vi "1-pointcal-v2.vi"() -> ()   [LabVIEW 2018]
uses:
  <vilib>/Utility/NIReport.llb/NI_report.lvclass
  <vilib>/Utility/NIReport.llb/Excel/NI_Excel.lvclass
  <vilib>/Utility/NIReport.llb/Report Type.ctl
  <vilib>/DAQmx/read.llb/DAQmx Read (Analog Wfm 1Chan NSamp).vi
  <vilib>/Utility/NIReport.llb/Append Text Table to Report (wrap).vi
  <vilib>/Utility/NIReport.llb/Append Numeric Table to Report (wrap).vi
  <vilib>/DAQmx/create/channels.llb/DAQmx Create Channel (AI-Voltage-Basic).vi
  <vilib>/DAQmx/configure/timing.llb/DAQmx Timing (Sample Clock).vi
  <vilib>/DAQmx/miscellaneous.llb/DAQmx Fill In Error Info.vi
  <vilib>/Utility/NIReport.llb/NI_ReportGenerationCore.lvlib
  <resource>/objmgr/daqmx.rc
panel:
  in  "Unit":enum16{"oz.in", "lbf-ft.", "lbf-in.", "N-m"}(ring)
  in  "Sensor ID:":tag
  in  "samples per channel":i32=4000
  in  "rate":dbl=500.0 format="%#_13g"
  in  "milliseconds to wait":u32=1000
  out "Cycles":i32=10
  out "Average":dbl[](array[numeric])=[2.9362440950071025]
  out "Template":refnum<class "NI_report.lvclass">
  out "Upper Limit":dbl=2.12
  out "Lower Limit":dbl=1.88
  out "output array":dbl[][](array[numeric])=[[3.9379769276696557, 2.0, 2.0, 3.7231645789771317, 3.939138075500426], [2.0, 2.0, 3.7939945966541258, 3.968166771269686, 2.0]]
  in  "stop":bool
  out "Torque":dbl=3.9379769276696557 format="%0.2f"
  out "Waveform Graph 2":waveform(dbl)(graph)={"t0"=timestamp(3654803301.2825823 s since 1904-01-01), "dt"=0.000333325, "Y"=array[6000 elements], "attributes"=variant("NI_ChannelName"=variant(string "6003/ai0"), "NI_UnitDescription"=variant(string "oz.in"))}
  in  "Continue":bool=TRUE
  out "Torque:":dbl=2.0
  in  "Humidity(%):":string="40"
  in  "Temp(F):":string="75"
  in  "FG Serial Number:":string="0211932-0056"
  in  "User Name:":string="Kyle Watts"
  in  "FG Model:":string(combo)="FG-40i"
  in  "Cal Dir:":string(combo)="CW"
  # "Calibration Tester"
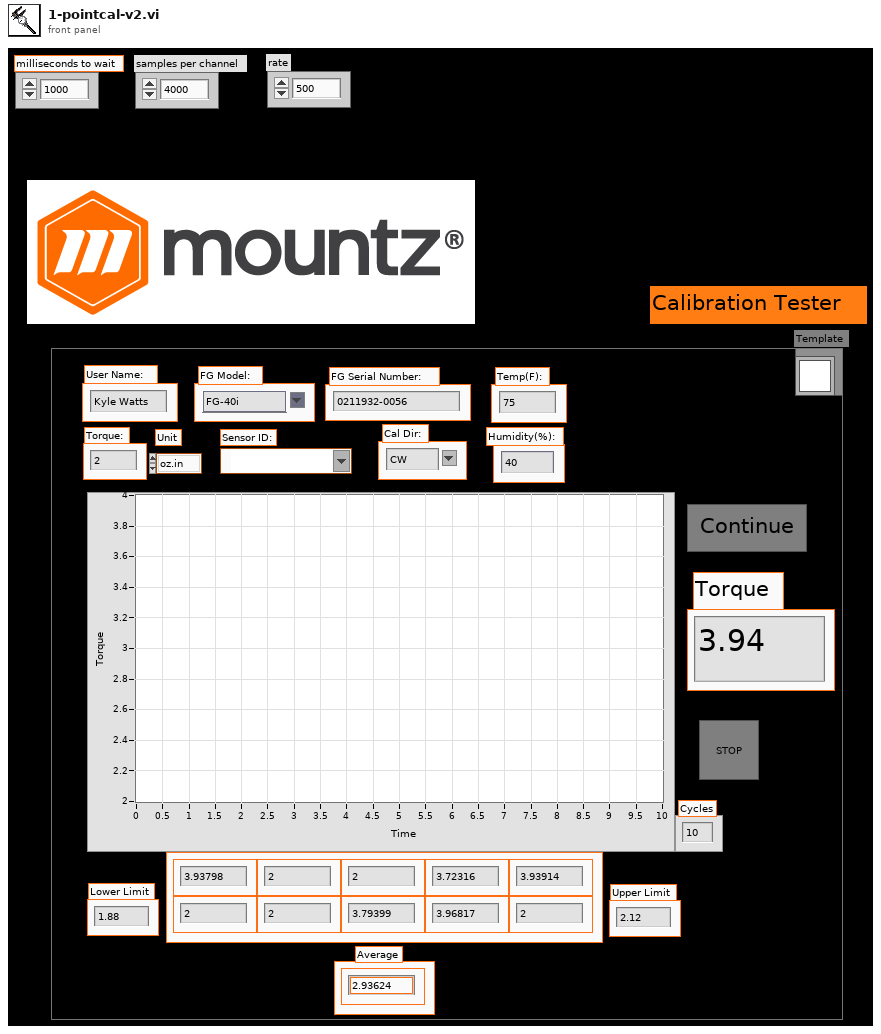
[diagram p1: front panel]
types:
  T1 = enum16{"Initialize ", "Set Torque", "Read Torque"}
  T2 = enum16{"Initialize ", "Set Torque", "Read Torque", "Save data"}
  T3 = cluster{"position (excel)":cluster{"row":i32, "column":i32}, "name (excel)":string, "bookmark (word)":string}
  T4 = cluster{"Charset (-1)":i16, "Weight (-1)":i16, "Name":string, "Size":string}
  T5 = typedef "NI_ReportGenerationCore.lvlib/Report Type.ctl" = enum16{"HTML", "Word", "Excel"}
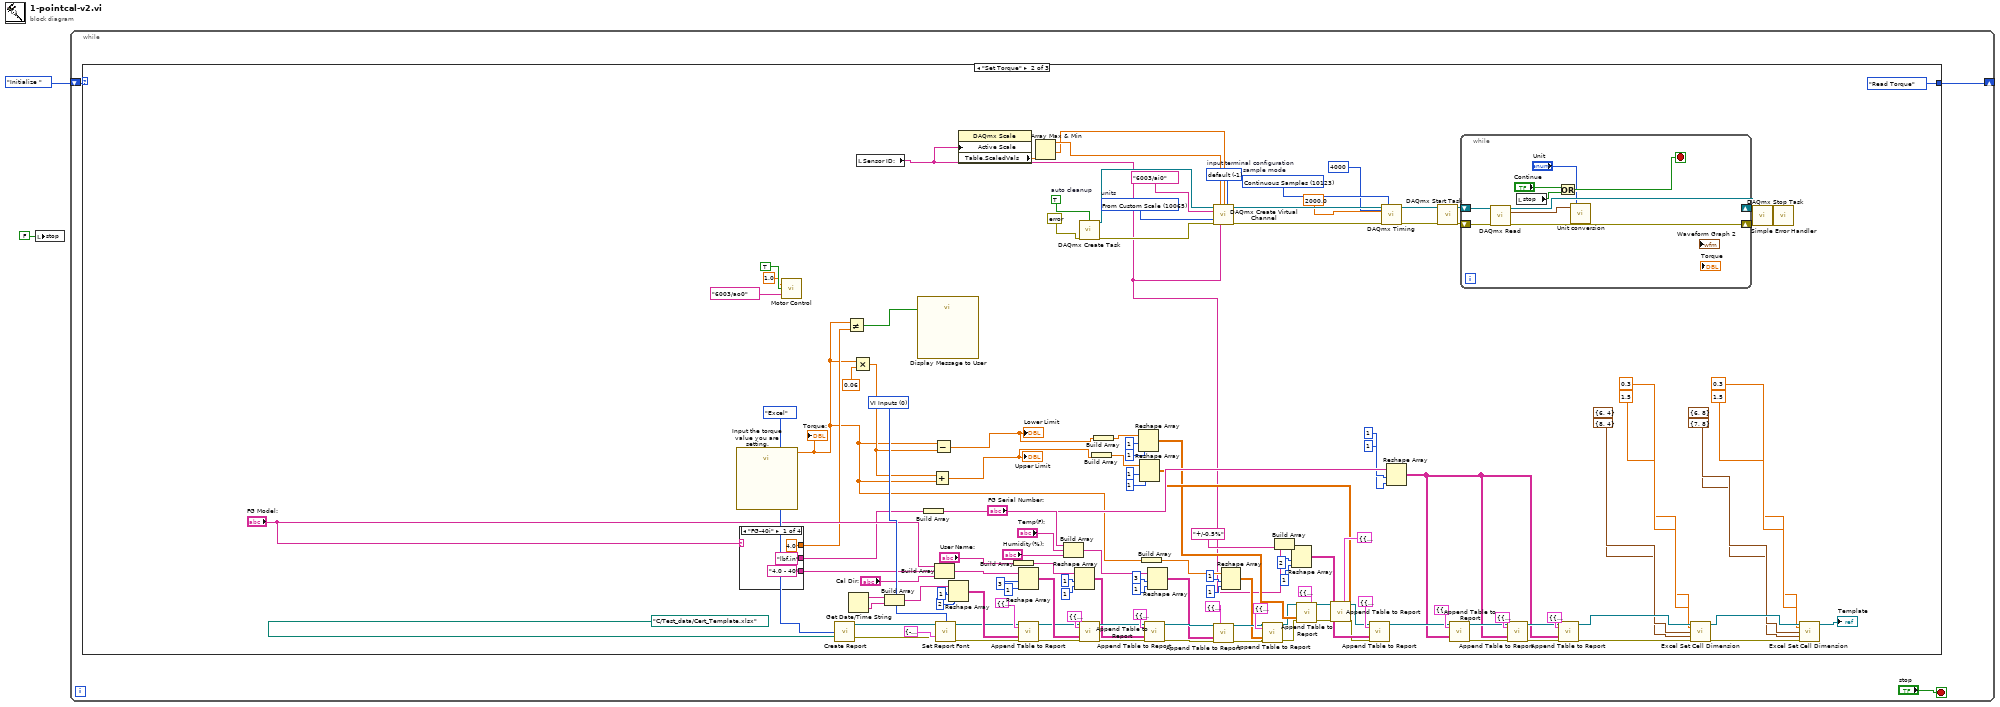
[diagram p0: block diagram]
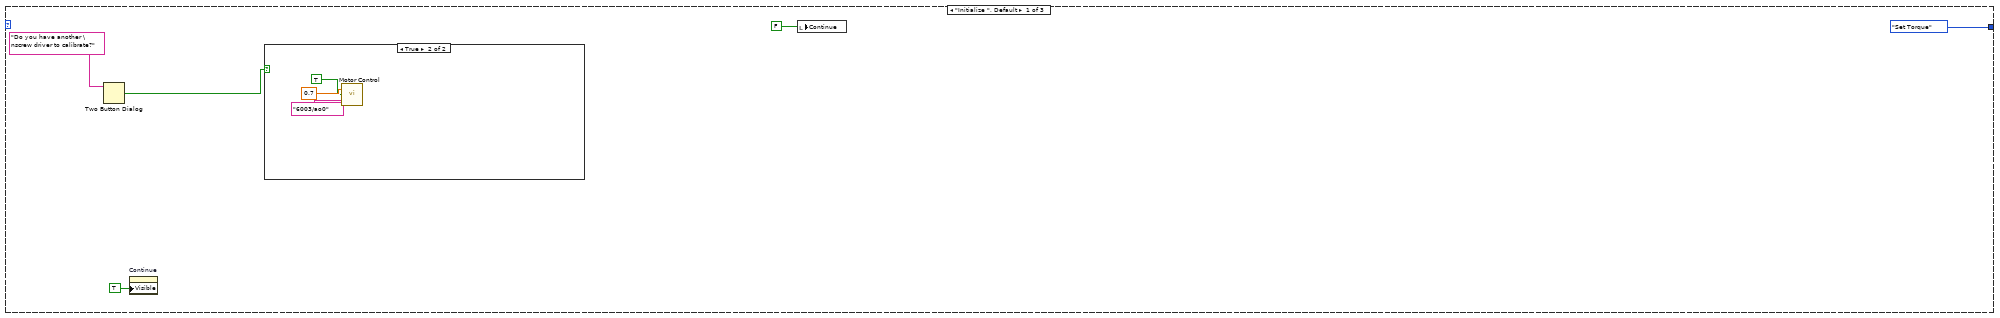
[diagram p2: hidden frame]
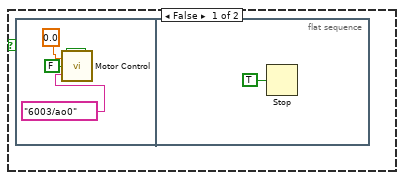
[diagram p3: hidden frame]
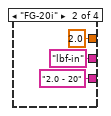
[diagram p4: hidden frame]
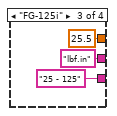
[diagram p5: hidden frame]
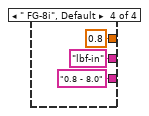
[diagram p6: hidden frame]
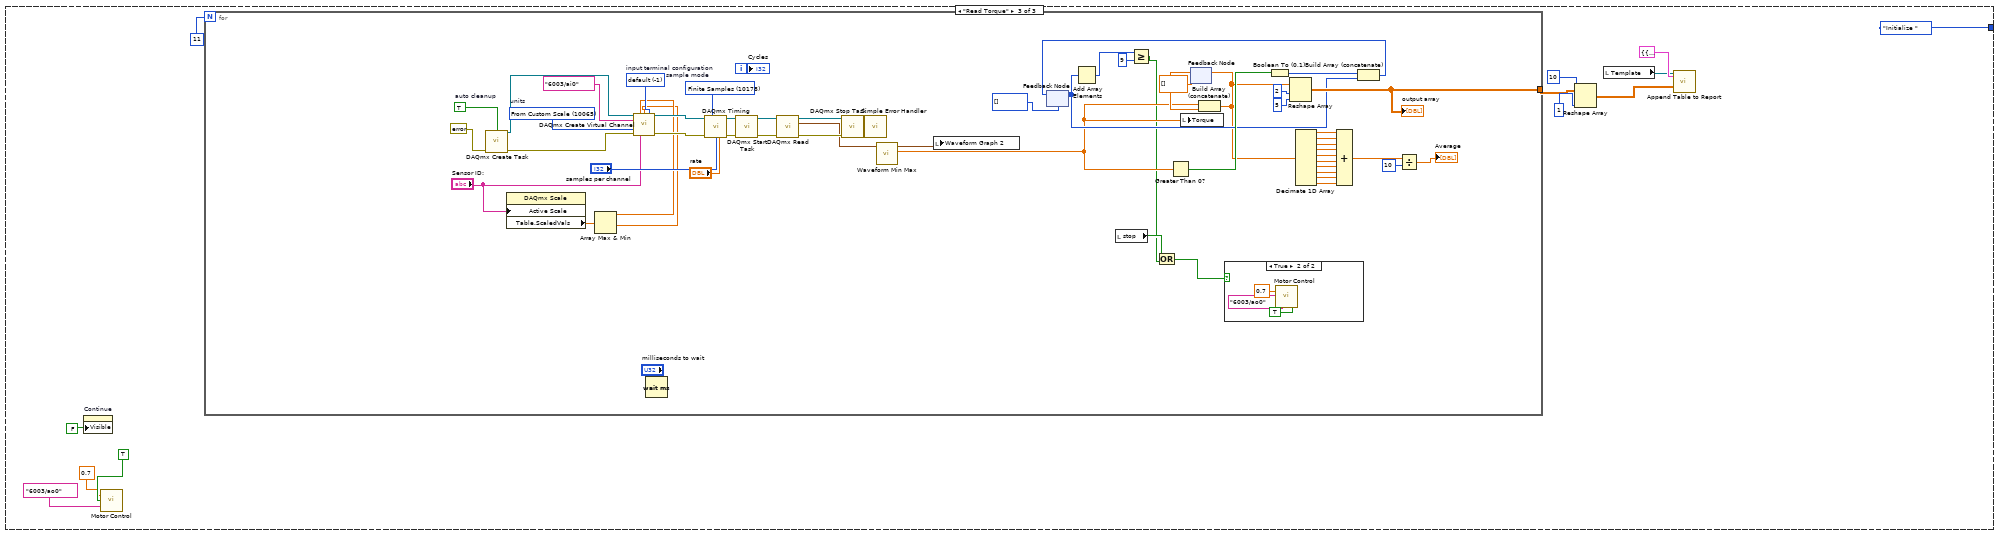
[diagram p7: hidden frame]
diagram:
  n1 = local write "stop"(FALSE ("stop")) -> ()
  n2 = while {
    shift-right: [w3] -> _
    shift-left: T1."Initialize " -> [w4]
    stop <- "stop" stop-if-true
    n3 = case shown="\"Set Torque\"" w4 {
      tunnel: [T2."Set Torque" T2."Read Torque" T2."Initialize "] -> w3
      frame "Initialize ", Default {
        n4 = Two Button Dialog(message="Do you have another \nscrew driver to calibrate?") -> (T button?=w6:bool)  [unwired: 2 in]
        n5 = property on="Continue" class="Bool (strict)"("Visible"=TRUE) -> ()  [unwired: 2 in, 2 out]
        n6 = case shown="True" w6 {
          frame False {
            n7 = flat-sequence {
              frame #0 {
                n8 = call "Motor Control.vi"("Run"=FALSE, "physical channels"=tag "6003/ao0", "Speed"=0.0) -> ()
              }
              frame #1 {
                n9 = Stop(stop? (T)=TRUE) -> ()
              }
            }
          }
          frame True {
            n10 = call "Motor Control.vi"("Run"=TRUE, "physical channels"=tag "6003/ao0", "Speed"=0.7) -> ()
          }
        }
        n11 = local write "Continue"(FALSE ("Continue")) -> ()
      }
      frame "Set Torque" {
        w54 = 10123 items=["Finite Samples"=10178, "Continuous Samples"=10123, "Hardware Timed Single Point"=12522]  # sample mode
        w52 = -1 items=["default"=-1, "RSE"=10083, "NRSE"=10078, "Differential"=10106, "Pseudodifferential"=12529]  # input terminal configuration
        w51 = 10065 items=["Volts"=10348, "From Custom Scale"=10065]  # units
        w48 = TRUE  # auto cleanup
        w120 = u16 0 items=["VI Inputs", "Font Dialog Box"] ("font settings source (VI Inputs)")
        n12 = call "Input the torque value you are setting."() -> ("Torque"=w63:dbl)  [unwired: 17 in, 2 out]
        "Torque:" <- w63
        n13 = case shown="\"FG-40i\"" "FG Model:" {
          tunnel: ["4.0 - 40" "2.0 - 20" "25 - 125" "0.8 - 8.0"] -> w99
          tunnel: ["lbf.in" "lbf-in" "lbf.in" "lbf-in"] -> w70
          tunnel: [4.0 2.0 25.5 0.8] -> w68
          frame "FG-40i" {
          }
          frame "FG-20i" {
          }
          frame "FG-125i" {
          }
          frame " FG-8i", Default {
          }
        }
        n14 = call "Motor Control.vi"("Run"=TRUE, "physical channels"=tag "6003/ao0", "Speed"=1.0) -> ()
        n15 = call <vilib>:"Create Report.vi"("report type"=Report_Type."Excel", "template (empty)"=path "C:/Test_data/Cert_Template.xlsx") -> ("report out"=w119:refnum<class "NI_report.lvclass">, "error out"=w118:errorcluster)  [unwired: 12 in]
        n16 = Not Equal?(x=w63, y=w68) -> (x != y?=w67:bool)
        n17 = Get Date/Time String() -> (date string=w137:string, time string=w138:string)  [unwired: 3 in]
        n18 = Multiply(x=w63, y=0.06) -> (x*y=w64:dbl)
        n19 = local read "Sensor ID:"() -> (w21:tag)
        n20 = Build Array(w137, w138) -> (w141:string[])
        n21 = call "Display Message to User"("Enable"=w67) -> ()  [unwired: 9 in, 2 out]
        n22 = Build Array(w70) -> (w73:string[])
        n23 = Add(x=w64, y=w63) -> (x+y=w30:dbl)
        "Upper Limit" <- w30
        n24 = Subtract(x=w63, y=w64) -> (x-y=w31:dbl)
        "Lower Limit" <- w31
        n25 = Build Array("FG Model:", w99, "Cal Dir:") -> (w101:string[])
        n26 = call-dynamic "Set Report Font.vi"("report in"=w119, "font settings source (VI Inputs)"=w120, "font settings"=T4 {"Charset (-1)"=-1, "Weight (-1)"=-1, "Name"="Calibri", "Size"=" 14"}, "error in (no error)"=w118) -> ("report out"=w116:refnum<class "NI_report.lvclass">, "error out"=w117:errorcluster)  [unwired: 9 in, 1 out]
        n27 = Reshape Array(w141, 1 ("dimension size"), 2 ("dimension size")) -> (w140:string[][])
        n28 = property class="DAQmx Scale"("Active Scale"=w21) -> ("Table.ScaledVals"=w20:dbl[])  [unwired: 2 in, 2 out]
        n29 = Build Array("User Name:") -> (w94:string[])
        n30 = Reshape Array(w101, 3 ("dimension size"), 1 ("dimension size")) -> (w100:string[][])
        n31 = call-poly <vilib>:"Append Table to Report.vi"("report in"=w116, "MS Office parameters"=T3 {"position (excel)"={"row"=4, "column"=8}, "name (excel)"="", "bookmark (word)"=""}, "text data"=w140, "error in (no error)"=w117) -> ("report out"=w96:refnum<class "NI_report.lvclass">, "error out"=w95:errorcluster)  [unwired: 8 in, 2 out]
        n32 = Array Max & Min(array=w20) -> (max value=w19:dbl, min value=w18:dbl)  [unwired: 2 out]
        n33 = Build Array("FG Serial Number:", "Temp(F):", "Humidity(%):") -> (w89:string[])
        n34 = Reshape Array(w94, 1 ("dimension size"), 1 ("dimension size")) -> (w90:string[][])
        n35 = call <vilib>:"DAQmx Create Task.vi"("auto cleanup"=w48, "error in"=errorcluster {"status"=FALSE, "code"=0, "source"=""}) -> ("task out"=w49:refnum<k21>, "error out"=w47:errorcluster)  [unwired: 12 in]
        n36 = call-poly <vilib>:"Append Table to Report.vi"("report in"=w96, "MS Office parameters"=T3 {"position (excel)"={"row"=5, "column"=1}, "name (excel)"="", "bookmark (word)"=""}, "text data"=w100, "error in (no error)"=w95) -> ("report out"=w131:refnum<class "NI_report.lvclass">, "error out"=w132:errorcluster)  [unwired: 8 in, 2 out]
        n37 = Build Array(w30) -> (w32:dbl[])
        n38 = Build Array(w31) -> (w33:dbl[])
        n39 = Reshape Array(w33, 1 ("dimension size"), 1 ("dimension size")) -> (w28:dbl[][])
        n40 = Reshape Array(w32, 1 ("dimension size"), 1 ("dimension size")) -> (w29:dbl[][])
        n41 = Build Array(w63) -> (w82:dbl[])
        n42 = call-poly <vilib>:"Append Table to Report.vi"("report in"=w131, "MS Office parameters"=T3 {"position (excel)"={"row"=5, "column"=4}, "name (excel)"="", "bookmark (word)"=""}, "text data"=w90, "error in (no error)"=w132) -> ("report out"=w130:refnum<class "NI_report.lvclass">, "error out"=w129:errorcluster)  [unwired: 8 in, 2 out]
        n43 = Reshape Array(w89, 3 ("dimension size"), 1 ("dimension size")) -> (w83:string[][])
        n44 = call-poly <vilib>:"DAQmx Create Virtual Channel.vi"("task in"=w49, "maximum value"=w19, "minimum value"=w18, "input terminal configuration"=w52, "physical channels"=tag "6003/ai0", "units"=w51, "error in"=w47, "custom scale name"=w21) -> ("task out"=w53:refnum<k21>, "error out"=w50:errorcluster)  [unwired: 6 in]
        n45 = call-poly <vilib>:"Append Table to Report.vi"("report in"=w130, "MS Office parameters"=T3 {"position (excel)"={"row"=5, "column"=8}, "name (excel)"="", "bookmark (word)"=""}, "text data"=w83, "error in (no error)"=w129) -> ("report out"=w127:refnum<class "NI_report.lvclass">, "error out"=w128:errorcluster)  [unwired: 8 in, 2 out]
        n46 = Reshape Array(w82, 1 ("dimension size"), 1 ("dimension size")) -> (w79:dbl[][])
        n47 = call-poly <vilib>:"Append Table to Report.vi"("report in"=w127, "MS Office parameters"=T3 {"position (excel)"={"row"=9, "column"=1}, "name (excel)"="", "bookmark (word)"=""}, "numerical data"=w79, "error in (no error)"=w128) -> ("report out"=w26:refnum<class "NI_report.lvclass">, "error out"=w27:errorcluster)  [unwired: 8 in, 2 out]
        n48 = Build Array(w21, "+/-0.5%") -> (w75:string[])
        n49 = Reshape Array(w75, 2 ("dimension size"), 1 ("dimension size")) -> (w74:string[][])
        n50 = call-poly <vilib>:"Append Table to Report.vi"("report in"=w26, "MS Office parameters"=T3 {"position (excel)"={"row"=9, "column"=4}, "name (excel)"="", "bookmark (word)"=""}, "numerical data"=w28, "error in (no error)"=w27) -> ("report out"=w25:refnum<class "NI_report.lvclass">, "error out"=w24:errorcluster)  [unwired: 8 in, 2 out]
        n51 = call-poly <vilib>:"Append Table to Report.vi"("report in"=w25, "MS Office parameters"=T3 {"position (excel)"={"row"=9, "column"=7}, "name (excel)"="", "bookmark (word)"=""}, "numerical data"=w29, "error in (no error)"=w24) -> ("report out"=w22:refnum<class "NI_report.lvclass">, "error out"=w23:errorcluster)  [unwired: 8 in, 2 out]
        n52 = call-poly <vilib>:"Append Table to Report.vi"("report in"=w22, "MS Office parameters"=T3 {"position (excel)"={"row"=7, "column"=4}, "name (excel)"="", "bookmark (word)"=""}, "text data"=w74, "error in (no error)"=w23) -> ("report out"=w126:refnum<class "NI_report.lvclass">)  [unwired: 8 in, 3 out]
        n53 = call-poly <vilib>:"DAQmx Timing.vi"("task/channels in"=w53, "sample mode"=w54, "samples per channel"=4000, "rate"=2000.0, "error in"=w50) -> ("task out"=w56:refnum<k21>, "error out"=w45:errorcluster)  [unwired: 9 in]
        n54 = Reshape Array(w73, 1 ("index"), 1 ("index")) -> (w69:string[][])
        n55 = call <vilib>:"DAQmx Start Task.vi"("task/channels in"=w56, "error in"=w45) -> ("task out"=w58:refnum<k21>, "error out"=w57:errorcluster)  [unwired: 12 in]
        n56 = call-poly <vilib>:"Append Table to Report.vi"("report in"=w126, "MS Office parameters"=T3 {"position (excel)"={"row"=9, "column"=2}, "name (excel)"="", "bookmark (word)"=""}, "text data"=w69) -> ("report out"=w125:refnum<class "NI_report.lvclass">, "error out"=w124:errorcluster)  [unwired: 9 in, 2 out]
        n57 = while {
          shift-right: [w156] -> w43
          shift-left: w58 -> [w158]
          shift-right: [w155] -> w42
          shift-left: w57 -> [w157]
          stop <- w152 stop-if-true
          n58 = call-poly <vilib>:"DAQmx Read.vi"("task/channels in"=w158, "error in"=w157) -> ("task out"=w156:refnum<k21>, "data"=w151:waveform(dbl), "error out"=w155:errorcluster)  [unwired: 11 in]
          n59 = local read "stop"() -> (w153:bool)
          n60 = Or(x="Continue", y=w153) -> (x .or. y?=w152:bool)
          n61 = call "Unit conversion.vi"("Convert to"="Unit", "Torque in (Nm)"=w151) -> ()  [unwired: 2 in, 2 out]
        }
        n62 = call-poly <vilib>:"Append Table to Report.vi"("report in"=w125, "MS Office parameters"=T3 {"position (excel)"={"row"=9, "column"=5}, "name (excel)"="", "bookmark (word)"=""}, "text data"=w69, "error in (no error)"=w124) -> ("report out"=w122:refnum<class "NI_report.lvclass">, "error out"=w123:errorcluster)  [unwired: 8 in, 2 out]
        n63 = call-poly <vilib>:"Append Table to Report.vi"("report in"=w122, "MS Office parameters"=T3 {"position (excel)"={"row"=9, "column"=8}, "name (excel)"="", "bookmark (word)"=""}, "text data"=w69, "error in (no error)"=w123) -> ("report out"=w115:refnum<class "NI_report.lvclass">, "error out"=w114:errorcluster)  [unwired: 8 in, 2 out]
        n64 = call <vilib>:"Excel Set Cell Dimension.vi"("report in"=w115, "width (-1)"=1.5, "height (-1)"=0.3, "start (-1, -1)"=cluster{"row":i32, "column":i32} {"row"=6, "column"=4}, "end (-1, -1)"=cluster{"row":i32, "column":i32} {"row"=8, "column"=4}, "error in (no error)"=w114) -> ("report out"=w109:refnum<class "NI_report.lvclass">, "error out"=w108:errorcluster)  [unwired: 8 in]
        n65 = call <vilib>:"DAQmx Stop Task.vi"("task/channels in"=w43, "error in"=w42) -> ("error out"=w41:errorcluster)  [unwired: 12 in, 1 out]
        n66 = call <vilib>:"Simple Error Handler.vi"("error in (no error)"=w41) -> ()  [unwired: 4 in, 5 out]
        n67 = call <vilib>:"Excel Set Cell Dimension.vi"("report in"=w109, "width (-1)"=1.5, "height (-1)"=0.3, "start (-1, -1)"=cluster{"row":i32, "column":i32} {"row"=6, "column"=8}, "end (-1, -1)"=cluster{"row":i32, "column":i32} {"row"=7, "column"=8}, "error in (no error)"=w108) -> ("report out"=→"Template":refnum<class "NI_report.lvclass">)  [unwired: 8 in, 1 out]
      }
      frame "Read Torque" {
        n68 = property on="Continue" class="Bool (strict)"("Visible"=FALSE) -> ()  [unwired: 2 in, 2 out]
        n69 = call "Motor Control.vi"("Run"=TRUE, "physical channels"=tag "6003/ao0", "Speed"=0.7) -> ()
        n70 = for {
          N: 11 -> [_]
          tunnel: [w239] -> w178
          i -> [w211]
          w196 = 10178 items=["Finite Samples"=10178, "Continuous Samples"=10123, "Hardware Timed Single Point"=12522]  # sample mode
          w193 = -1 items=["default"=-1, "RSE"=10083, "NRSE"=10078, "Differential"=10106, "Pseudodifferential"=12529]  # input terminal configuration
          w191 = 10065 items=["Volts"=10348, "From Custom Scale"=10065]  # units
          w190 = TRUE  # auto cleanup
          n71 = call <vilib>:"DAQmx Create Task.vi"("auto cleanup"=w190, "error in"=errorcluster {"status"=FALSE, "code"=0, "source"=""}) -> ("task out"=w202:refnum<k21>, "error out"=w201:errorcluster)  [unwired: 12 in]
          n72 = property class="DAQmx Scale"("Active Scale"="Sensor ID:") -> ("Table.ScaledVals"=w185:dbl[])  [unwired: 2 in, 2 out]
          n73 = Array Max & Min(array=w185) -> (max value=w184:dbl, min value=w183:dbl)  [unwired: 2 out]
          n74 = call-poly <vilib>:"DAQmx Create Virtual Channel.vi"("task in"=w202, "maximum value"=w184, "minimum value"=w183, "input terminal configuration"=w193, "physical channels"=tag "6003/ai0", "units"=w191, "error in"=w201, "custom scale name"="Sensor ID:") -> ("task out"=w204:refnum<k21>, "error out"=w203:errorcluster)  [unwired: 6 in]
          n75 = Wait (ms)(milliseconds to wait="milliseconds to wait") -> ()  [unwired: 1 out]
          n76 = call-poly <vilib>:"DAQmx Timing.vi"("task/channels in"=w204, "sample mode"=w196, "samples per channel"="samples per channel", "rate"="rate", "error in"=w203) -> ("task out"=w205:refnum<k21>, "error out"=w200:errorcluster)  [unwired: 9 in]
          n77 = call <vilib>:"DAQmx Start Task.vi"("task/channels in"=w205, "error in"=w200) -> ("task out"=w207:refnum<k21>, "error out"=w206:errorcluster)  [unwired: 12 in]
          n78 = call-poly <vilib>:"DAQmx Read.vi"("task/channels in"=w207, "error in"=w206) -> ("task out"=w199:refnum<k21>, "data"=w188:waveform(dbl), "error out"=w198:errorcluster)  [unwired: 11 in]
          n79 = call <vilib>:"DAQmx Stop Task.vi"("task/channels in"=w199, "error in"=w198) -> ("error out"=w197:errorcluster)  [unwired: 12 in, 1 out]
          n80 = call <vilib>:"Simple Error Handler.vi"("error in (no error)"=w197) -> ()  [unwired: 4 in, 5 out]
          n81 = call <vilib>:"Waveform Min Max.vi"("waveform in"=w188) -> ("Y max"=w214:dbl, "waveform out"=w213:waveform(dbl))  [unwired: 5 in, 4 out]
          n82 = local write "Waveform Graph 2"(w213) -> ()
          n83 = feedback #1(i16[] []) -> (w234:i16[])
          n84 = Add Array Elements(numeric array=w234) -> (sum=w236:i16)
          n85 = local read "stop"() -> (w212:bool)
          n86 = Greater Or Equal?(x=w236, y=i16 9) -> (x >= y?=w187:bool)
          n87 = Or(x=w212, y=w187) -> (x .or. y?=w210:bool)
          n88 = Greater Than 0?(x=w214) -> (x > 0?=w238:bool)
          n89 = local write "Torque"(w214) -> ()
          n90 = feedback #2(dbl[] []) -> (w231:dbl[])
          n91 = Build Array (concatenate)(w214, w231) -> (w227:dbl[])
          n92 = feedback-in #2(w227) -> ()
          n93 = case shown="True" w210 {
            frame False {
            }
            frame True {
              n94 = call "Motor Control.vi"("Run"=TRUE, "physical channels"=tag "6003/ao0", "Speed"=0.7) -> ()
            }
          }
          n95 = Boolean To (0,1)(Boolean=w238) -> (0, 1=w237:i16)
          n96 = Reshape Array(w227, 2 ("dimension size"), 5 ("dimension size")) -> (w239:dbl[][])
          "output array" <- w239
          n97 = Decimate 1D Array(w227) -> (w226:dbl[], w225:dbl[], w224:dbl[], w223:dbl[], w222:dbl[], w221:dbl[], w220:dbl[], w219:dbl[], w218:dbl[], w217:dbl[])
          n98 = Compound Arithmetic op=ADD(w226, w225, w224, w223, w222, w221, w220, w219, w218, w217) -> (w209:dbl[])
          n99 = Build Array (concatenate)(w237, w234) -> (w235:i16[])
          n100 = feedback-in #1(w235) -> ()
          n101 = Divide(x=w209, y=10) -> (x/y=→"Average":dbl[])
          "Cycles" <- w211
        }
        n102 = Reshape Array(w178, 10 ("dimension size"), 1 ("dimension size")) -> (w177:dbl[][])
        n103 = local read "Template"() -> (w175:refnum<class "NI_report.lvclass">)
        n104 = call-poly <vilib>:"Append Table to Report.vi"("report in"=w175, "MS Office parameters"=T3 {"position (excel)"={"row"=13, "column"=1}, "name (excel)"="", "bookmark (word)"=""}, "numerical data"=w177) -> ()  [unwired: 9 in, 4 out]
      }
    }
  }
